vi "getILCCommunications.vi"(11 "Model in":refnum<class "Model.lvclass">) -> (2 "ILCCommunications":refnum<class "ILCCommunications.lvclass">, 3 "Model out":refnum<class "Model.lvclass">)   [LabVIEW 2016, in "Model.lvclass"]
uses:
  Model.lvclass
  ILCCommunications/ILCCommunications.lvclass
  Model.lvclass/Model.ctl
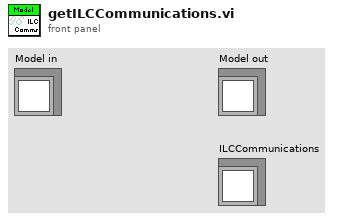
[diagram p1: front panel]
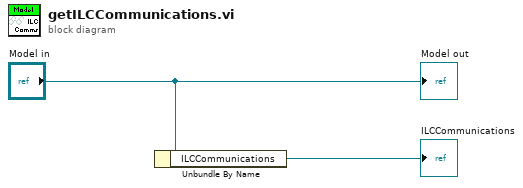
[diagram p0: block diagram]
diagram:
  n1 = Unbundle By Name("Model in") -> ("ILCCommunications"=→"ILCCommunications":refnum<class "ILCCommunications.lvclass">)
  "Model out" <- "Model in"
